vi "Add SIM Profile.vi"(8 "error in (no error)":errorcluster, 10 "SIM Profile Name (\"SIM1\")":string="SIM1", 11 "VISA resource name":refnum<visa-resource-name>) -> (0 "error out":errorcluster, 3 "VISA resource name out":refnum<visa-resource-name>)   [LabVIEW 2020, in "Rohde&Schwarz CMXP Base.lvlib"]
doc: "Creates a SIM profile with the specified name.\n\nAssign a unique name to each named object within the test environment. Assigning an already used name can be rejected with an error message, even if the other object has not the same type as the new object.\n\nAttribute:\nRSCMXPBASE_ATTR_SIM_PROFILE_ADD\n\nRemote-control command:\nCREate:SIMProfile"
uses:
  <instrlib>/Rohde&Schwarz CMXP Base/Rohde&Schwarz CMXP Base.lvlib
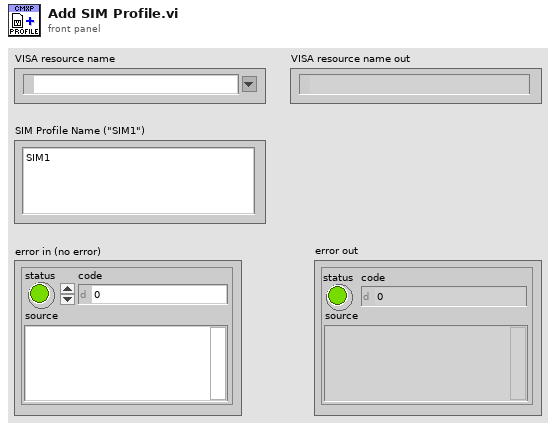
[diagram p1: front panel]
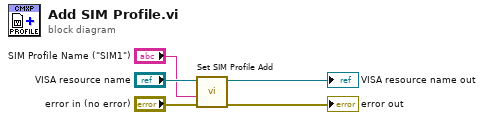
[diagram p0: block diagram]
diagram:
  n1 = call "Set SIM Profile Add"("error in (no error)"="error in (no error)", "SIM Profile Add ()"="SIM Profile Name (\"SIM1\")", "instrument handle"="VISA resource name") -> ("error out"=→"error out":errorcluster, "instrument handle out"=→"VISA resource name out":refnum<visa-resource-name>)  [unwired: 7 in]
